vi "Open Session.vi"(0 "fpga in":refnum<k20>, 7 "emulation model":T1=enum."PXIe-5170R (8CH)", 11 "error in":errorcluster) -> (4 "device session out":refnum<class "Device Session.lvclass">, 15 "error out":errorcluster)   [LabVIEW 2015, in "Device Session.lvclass"]
doc: "Opens a session to all bundled design libraries, including Register Bus, Multirecord Acquisition, Configuration, and Calibration, and initializes the scaling coefficients. This VI bundles these into a DVR session and wraps it with the session class wrapper.\n\n<B>Input Parameters</B>\n\n<B>fpga reference in</B> is the reference to the FPGA VI or bitfile of the RIO device specified. This parameter is obtained from the 'Open FPGA Reference' VI of this library.\n\n<B>sample fifo size (bytes)</B> is the size of the FIFO that will be used to store acquired samples.\n\n<B>error in</B> describes error conditions that occur before this node runs. This input provides standard 'error in' functionality.\n\n<B>Output Parameters</B>\n\n<B>device session out</B> passes a reference to the session to the next VI.\n\n<B>error out</B> contains error information. This output provides standard 'error out' functionality."
uses:
  Device Session.lvclass
  <instrlib>/HSAI-RIO/Types/v1/Host/Typedefs/Model Name.ctl
  Private/Typedef/Device Session Object.ctl
  FPGA Refnum.ctl
  <instrlib>/HSAI-RIO/Config/Interface/v1/Host/niHSAI Config v1 Host.lvclass
  <instrlib>/HSAI-RIO/Types/v1/Host/Typedefs/Channel Configuration.ctl
  <instrlib>/HSAI-RIO/Types/v1/Host/Typedefs/Coupling.ctl
  <instrlib>/HSAI-RIO/Types/v1/Host/Typedefs/Impedance.ctl
  <instrlib>/HSAI-RIO/Types/v1/Host/Typedefs/Bandwidth.ctl
  Device Session.lvclass/Device Session.ctl
  <instrlib>/HSAI-RIO/Config/Interface/v1/Host/Protected/Configure ADC Clock For Onboard.vi
  <instrlib>/_niInstr/FIFO Register Bus/v1/Host/niInstr FIFO Register Bus v1 Host.lvclass
  <instrlib>/HSAI-RIO/Config/Group A/v1/Host/Main/niHSAI Group A Config v1 Host.lvclass
  <instrlib>/_niInstr/Instruction Framework/v1/Host/Subsystem Map/niInstr Subsystem Map v1 Host.lvclass
  <instrlib>/HSAI-RIO/Cal Data/Group A/v1/Host/Cal Data/niHSAI Group A Cal Data v1 Host.lvclass
  <instrlib>/HSAI-RIO/Types/v1/Host/niHSAI Types v1 Host.lvlib
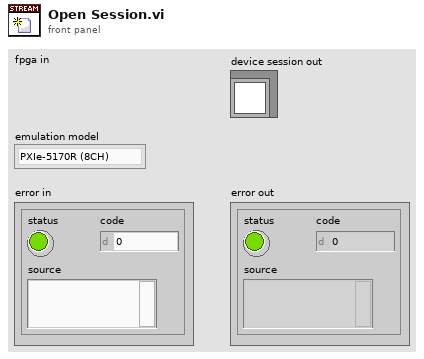
[diagram p1: front panel]
types:
  T1 = typedef "niHSAI Types v1 Host.lvlib/Model Name.ctl" = enum8{"None", "PXIe-5170R (4CH)", "PXIe-5170R (8CH)", "PXIe-5171R (8CH)"}
  T2 = typedef "Device Session.lvclass/Device Session Object.ctl" = cluster{"ni5171R FPGA Reference":T3, "niHSAI config":refnum<class "niHSAI Config v1 Host.lvclass">, "configured scaling coefficients":cluster{"gain":dbl, "offset":dbl}[], "number of channels to stream":u8, "selected acq channels":bool[], "number of channels":u32, "actual channel configuration":T4[], "configured channels":bool[], "sample clock rate (Hz)":dbl}
  T3 = typedef "Device Session.lvclass/FPGA Refnum.ctl" = refnum<k20>
  T4 = typedef "niHSAI Types v1 Host.lvlib/Channel Configuration.ctl" = cluster{"channel":u32, "coupling":T5, "impedance":T6, "bandwidth":T7, "vertical range":dbl, "vertical offset":dbl}
  T5 = typedef "niHSAI Types v1 Host.lvlib/Coupling.ctl" = enum8{"Default", "DC", "AC"}
  T6 = typedef "niHSAI Types v1 Host.lvlib/Impedance.ctl" = enum8{"Default", "1 mega ohm", "50 ohm"}
  T7 = typedef "niHSAI Types v1 Host.lvlib/Bandwidth.ctl" = enum8{"Default", "Full Bandwidth", "Anti-alias Filter"}
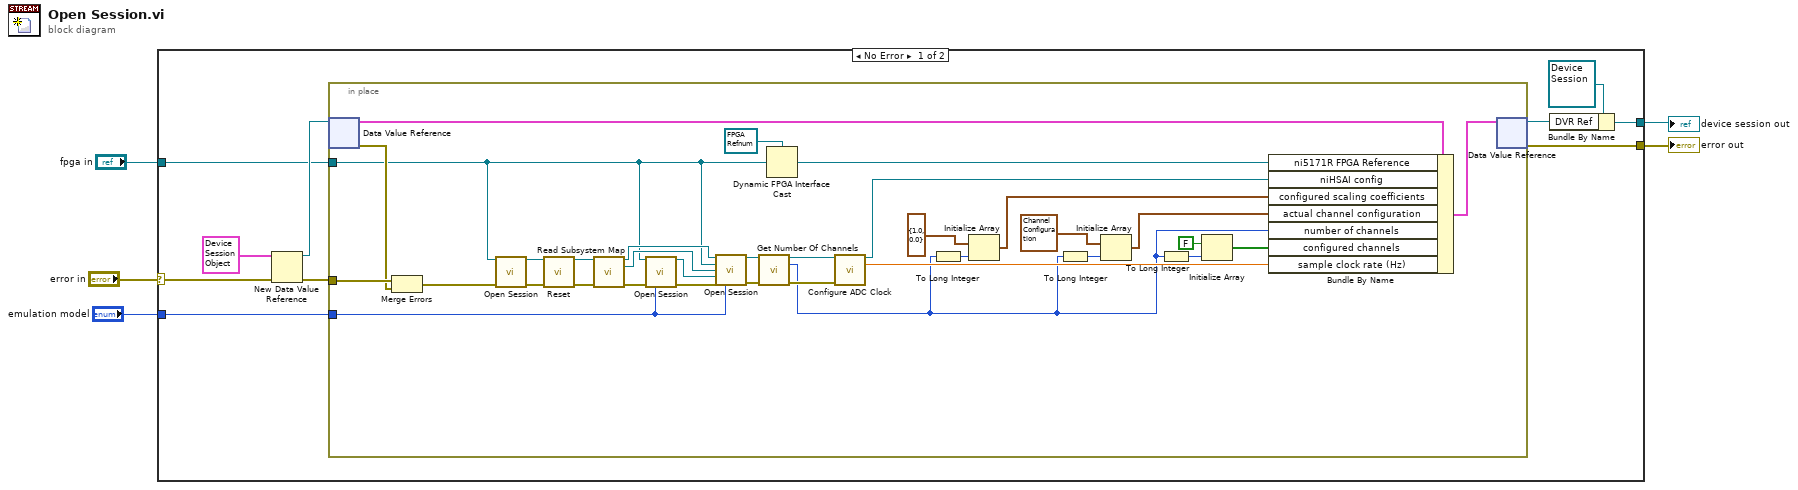
[diagram p0: block diagram]
diagram:
  n1 = case shown="No Error" "error in" {
    selector: "error in" -> [w13 w50]
    tunnel: [w7 w50] -> w4
    tunnel: [w14 _] -> w3
    tunnel: "fpga in" -> [w6 _]
    tunnel: "emulation model" -> [w8 _]
    frame No Error {
      n2 = New Data Value Reference(data value=T2 {"ni5171R FPGA Reference"=refnum, "niHSAI config"=refnum, "configured scaling coefficients"=[], "number of channels to stream"=0, "selected acq channels"=[], "number of channels"=0, "actual channel configuration"=[], "configured channels"=[], "sample clock rate (Hz)"=0.0} ("Cluster of class private data"), error in=w13) -> (data value reference=w10:refnum<data-value>, error out=w12:errorcluster)
      n3 = in-place {
        in-place-border: w12 -> [w37]
        in-place-border: w6 -> [w28]
        in-place-border: w8 -> [w16]
        n4 = in-place-dvr #1(w10) -> (w35:T2, w36:errorcluster)
        n5 = Merge Errors(w37, w36) -> (w27:errorcluster)
        n6 = call <instrlib>:"Open Session.vi"("fpga ref"=w28, "error in"=w27) -> ("session out"=w49:refnum<class "niInstr FIFO Register Bus v1 Host.lvclass">, "error out"=w42:errorcluster)  [unwired: 12 in]
        n7 = call-dynamic "Reset.vi"("session in"=w49, "error in"=w42) -> ("session out"=w48:refnum<class "niInstr FIFO Register Bus v1 Host.lvclass">, "error out"=w41:errorcluster)  [unwired: 12 in]
        n8 = call <instrlib>:"Read Subsystem Map.vi"("instruction target in"=w48, "error in"=w41) -> ("instruction target out"=w43:refnum<class "niInstr FIFO Register Bus v1 Host.lvclass">, "subsystem map"=w44:refnum<class "niInstr Subsystem Map v1 Host.lvclass">, "error out"=w47:errorcluster)  [unwired: 11 in]
        n9 = call <instrlib>:"Open Session.vi"("fpga reference"=w28, "error in"=w47, "emulation model name"=w16) -> ("session out"=w45:refnum<class "niHSAI Group A Cal Data v1 Host.lvclass">, "error out"=w46:errorcluster)  [unwired: 11 in]
        n10 = call <instrlib>:"Open Session.vi"("register bus in"=w43, "fpga interface in"=w28, "subsystem map in"=w44, "calibration data in"=w45, "error in"=w46, "emulation model name"=w16) -> ("session out"=w38:refnum<class "niHSAI Group A Config v1 Host.lvclass">, "error out"=w39:errorcluster)  [unwired: 8 in]
        n11 = call-dynamic "Get Number Of Channels.vi"("session in"=w38, "error in"=w39) -> ("session out"=w26:refnum<class "niHSAI Group A Config v1 Host.lvclass">, "number of channels"=w21:u32, "error out"=w25:errorcluster)  [unwired: 11 in]
        n12 = Dynamic FPGA Interface Cast(Session In=T3 refnum ("FPGA Interface"), Type=w28) -> (Session Out=w29:T3)
        n13 = call-poly <instrlib>:"Configure ADC Clock.vi"("session in"=w26, "error in"=w25) -> ("session out"=w17:refnum<class "niHSAI Group A Config v1 Host.lvclass">, "actual adc clock rate (Hz)"=w24:dbl)  [unwired: 9 in, 3 out]
        n14 = To Long Integer(number=w21) -> (32bit integer=w23:i32)
        n15 = Initialize Array(cluster{dbl, dbl} {1.0, 0.0}, w23) -> (w18:cluster{dbl, dbl}[])
        n16 = To Long Integer(number=w21) -> (32bit integer=w22:i32)
        n17 = Initialize Array(T4 {"channel"=0, "coupling"=enum."Default", "impedance"=enum."Default", "bandwidth"=enum."Default", "vertical range"=0.0, "vertical offset"=0.0} ("channel configuration"), w22) -> (w19:T4[])
        n18 = To Long Integer(number=w21) -> (32bit integer=w31:i32)
        n19 = Initialize Array(FALSE, w31) -> (w32:bool[])
        n20 = Bundle By Name(cluster=w35, "ni5171R FPGA Reference"=w29, "niHSAI config"=w17, "configured scaling coefficients"=w18, "actual channel configuration"=w19, "number of channels"=w21, "configured channels"=w32, "sample clock rate (Hz)"=w24) -> (w34:T2)
        n21 = in-place-dvr #1(w34) -> (w9:refnum<data-value>, w7:errorcluster)
      }
      n22 = Bundle By Name(cluster=refnum<class "Device Session.lvclass"> refnum ("Device Session.lvclass"), "DVR Ref"=w9) -> (w14:refnum<class "Device Session.lvclass">)
    }
    frame Error {
    }
  }
  "error out" <- w4
  "device session out" <- w3
